vi "test_TimeOut Error.vi"(8 "error in (no error)":errorcluster, 11 "TestCase in":refnum<class "Instrument Addon Host API Tests.lvclass">) -> (0 "error out":errorcluster, 3 "TestCase out":refnum<class "Instrument Addon Host API Tests.lvclass">)   [LabVIEW 2018, in "Instrument Addon Host API Tests.lvclass"]
uses:
  Instrument Addon Host API Tests.lvclass
  Addon/Addon Shared/Types/Buffered RT Instrument Command.ctl
  Addon/Addon Shared/Types/Response Wait Type.ctl
  <vilib>/addons/_JKI Toolkits/VI Tester/TestCase.llb/TestCase.lvclass
  APIs/Host Automation API/Instrument Host Automation API.lvlib
  Addon/Addon Shared/Instrument Addon Shared.lvlib
  C:/Program Files (x86)/National Instruments/LabVIEW 2018/vi.lib/addons/_JKI Toolkits/VI Tester/TestCase.llb/TestCase.lvclass
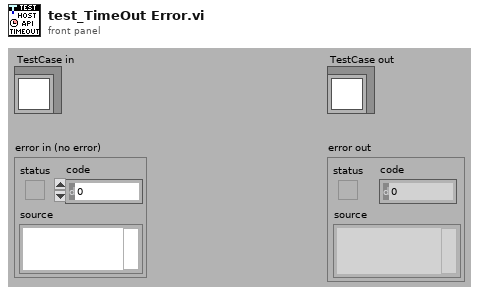
[diagram p1: front panel]
types:
  T1 = typedef "Instrument Addon Shared.lvlib/Buffered RT Instrument Command.ctl" = cluster{"Command":string, "Response Expected?":bool, "Wait Type":T2, "Wait Value":dbl}
  T2 = typedef "Instrument Addon Shared.lvlib/Response Wait Type.ctl" = enum16{"Byte Count", "Wait sec"}
  T3 = typedef "NI STM.lvlib/TCP Connection Info.ctl" = cluster{"connection ID":refnum<k5>, "meta data":T4[]}
  T4 = typedef "NI STM.lvlib/MetaDataElement.ctl" = string
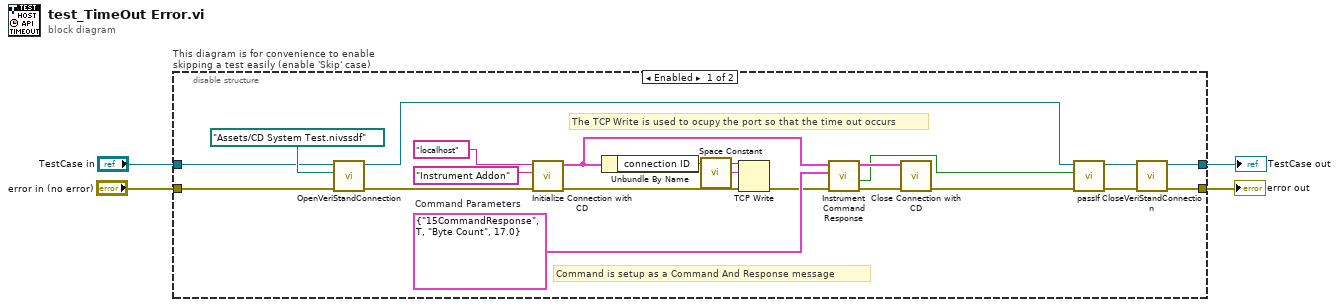
[diagram p0: block diagram]
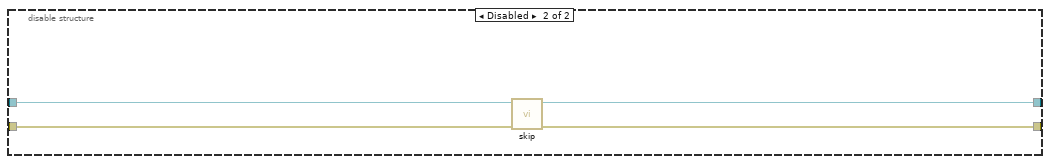
[diagram p2: hidden frame]
diagram:
  n1 = disable-structure "This diagram is for convenience to enable skipping a test easily (enable 'Skip' case)" shown="Enabled" {
    disable-tunnel: "TestCase in" -> [w21 w29]
    disable-tunnel: [w19 w27] -> w1
    disable-tunnel: [w20 w28] -> w3
    disable-tunnel: "error in (no error)" -> [w22 w26]
    frame Enabled {
      w7 = T1 {"Command"="15CommandResponse", "Response Expected?"=TRUE, "Wait Type"=enum."Byte Count", "Wait Value"=17.0}  # Command Parameters
      # "The TCP Write is used to ocupy the port so that the time out occurs"
      # "Command is setup as a Command And Response message"
      n2 = call-dynamic "OpenVeriStandConnection.vi"("error in (no error)"=w22, "System Definition File"=path "Assets/CD System Test.nivssdf", "VeriStand Test Case in"=w21) -> ("error out"=w18:errorcluster, "VeriStand Test Case out"=w12:refnum<class "Instrument Addon Host API Tests.lvclass">)  [unwired: 6 in, 1 out]
      n3 = call "Initialize Connection with CD.vi"("error in (no error)"=w18, "TCP Service"="Instrument Addon", "IP Address"="localhost") -> ("error out"=w6:errorcluster, "connection info out"=w11:T3)  [unwired: 7 in]
      n4 = Unbundle By Name(w11) -> ("connection ID"=w10:refnum<k5>)
      n5 = call <vilib>:"Space Constant.vi"() -> ("String"=w8:string)
      n6 = TCP Write(connection ID=w10, data in=w8, error in (no error)=w6) -> (error out=w5:errorcluster)  [unwired: 1 in, 2 out]
      n7 = call "Instrument Command Response.vi"("error in (no error)"=w5, "Command Parameters"=w7, "Comm.Info"=w11) -> ("error out"=w14:errorcluster, "Timed Out?"=w9:bool, "Comm.Info"=w13:T3)  [unwired: 5 in, 1 out]
      n8 = call "Close Connection with CD.vi"("error in"=w14, "Comm.Info"=w13) -> ("error out"=w15:errorcluster)  [unwired: 9 in]
      n9 = call-dynamic "passIf.vi"("error in (no error)"=w15, "pass"=w9, "TestCase in"=w12) -> ("error out"=w17:errorcluster, "TestCase out"=w16:refnum<class "Instrument Addon Host API Tests.lvclass">)  [unwired: 7 in]
      n10 = call-dynamic "CloseVeriStandConnection.vi"("error in (no error)"=w17, "VeriStand Test Case in"=w16) -> ("error out"=w20:errorcluster, "VeriStand Test Case out"=w19:refnum<class "Instrument Addon Host API Tests.lvclass">)  [unwired: 8 in]
    }
    frame Disabled {
      # "skip test result while test is under development"
      n11 = call <vilib>:"skip.vi"("error in (no error)"=w26, "TestCase in"=w29) -> ("error out"=w28:errorcluster, "TestCase out"=w27:refnum<class "Instrument Addon Host API Tests.lvclass">)  [unwired: 8 in]
    }
  }
  "error out" <- w3
  "TestCase out" <- w1
